vi "scan COM ports for XYZ stage.vi"(8 "error in (no error)":errorcluster) -> (0 "error out":errorcluster, 1 "Stage found?":bool, 2 "card type (F for old cards, T for new cards)":bool, 3 "VISA resource name out":refnum<visa-resource-name>)   [LabVIEW 2012]
uses:
  <vilib>/Instr/_visa.llb/VISA Flush IO Buffer Mask.ctl
  <vilib>/Instr/_visa.llb/VISA Find Search Mode.ctl
  <vilib>/Instr/_visa.llb/VISA Configure Serial Port (Instr).vi
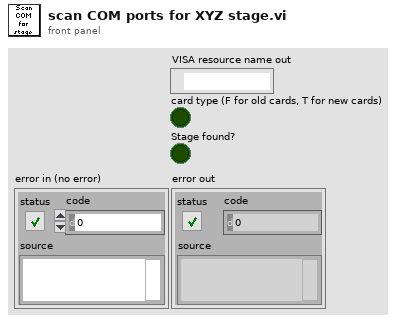
[diagram p1: front panel]
types:
  T1 = typedef "VISA Find Search Mode.ctl" = u32
  T2 = typedef "VISA Flush IO Buffer Mask.ctl" = u16
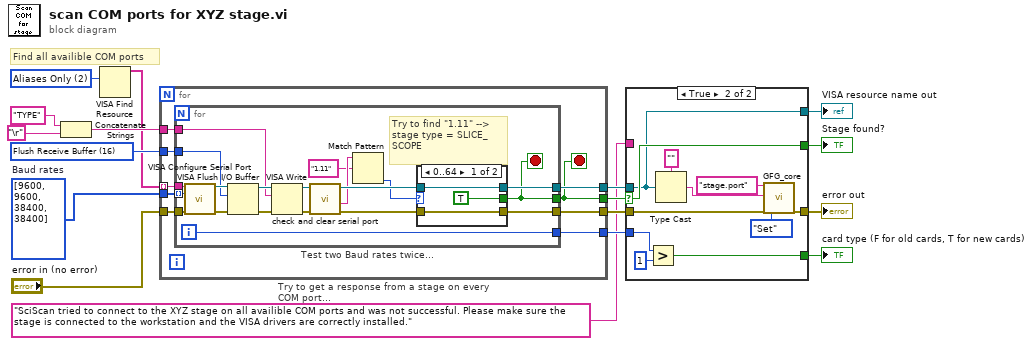
[diagram p0: block diagram]
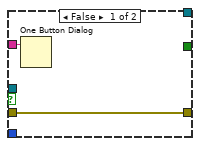
[diagram p2: hidden frame]
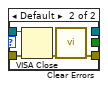
[diagram p3: hidden frame]
diagram:
  w13 = T1 2 items=["Canonical Names Only"=0, "Aliases Only"=2, "Include Matching Aliases"=3, "Include All Aliases"=4] ("Search Mode")
  w12 = u32[] [9600, 9600, 38400, 38400]  # Baud rates
  w16 = T2 16 items=["Flush Receive Buffer"=16, "Write Transmit Buffer to Device"=32, "Flush Receive Buffer (No I/O)"=64, "Flush Transmit Buffer"=128] ("Mask")
  # "Find all availible COM ports"
  n1 = Concatenate Strings("TYPE" ("write buffer"), "\r") -> (w14:string)
  n2 = VISA Find Resource(10:w13) -> (3:w11:string[])  [unwired: 2 in, 2 out]
  n3 = for "Try to get a response from a stage on every COM port..." {
    tunnel: w11 -> [w26] mode=indexing
    tunnel: w16 -> [w25]
    tunnel: w14 -> [w24]
    tunnel: w12 -> [w23]
    tunnel: [w22] -> w6
    tunnel: [w21] -> w5
    tunnel: [w20] -> w7
    tunnel: [w19] -> w9
    tunnel: "error in (no error)" -> [w18]
    stop <- w20 stop-if-true
    n4 = for "Test two Baud rates twice..." {
      tunnel: w26 -> [w40]
      tunnel: w25 -> [w37]
      tunnel: w24 -> [w36]
      tunnel: [w35] -> w22
      tunnel: [w34] -> w21
      tunnel: w23 -> [w33] mode=indexing
      tunnel: [w32] -> w19
      tunnel: [w31] -> w20
      tunnel: w18 -> [w30]
      i -> [w32]
      stop <- w31 stop-if-true
      # "Try to find \"1.11\" --> stage type = SLICE_SCOPE"
      n5 = call-poly "VISA Configure Serial Port"("VISA resource name"=w40, "baud rate (9600)"=w33, "error in (no error)"=w30) -> ("VISA resource name out"=w45:refnum<visa-resource-name>, "error out"=w46:errorcluster)  [unwired: 11 in]
      n6 = VISA Flush I/O Buffer(VISA resource name=w45, mask (16)=w37, error in (no error)=w46) -> (VISA resource name out=w39:refnum<visa-resource-name>, error out=w38:errorcluster)
      n7 = VISA Write(VISA resource name=w39, write buffer=w36, error in (no error)=w38) -> (VISA resource name out=w44:refnum<visa-resource-name>, error out=w43:errorcluster)  [unwired: 1 out]
      n8 = call "check and clear serial port.vi"("error in (no error)"=w43, "VISA resource name in"=w44) -> ("error out"=w41:errorcluster, "read buffer"=w28:string, "VISA resource name out"=w42:refnum<visa-resource-name>)  [unwired: 6 in, 1 out]
      n9 = Match Pattern(string=w28, regular expression="1.11" ("read buffer")) -> (offset past match=w29:i32)  [unwired: 1 in, 3 out]
      n10 = case shown="0..64" w29 {
        tunnel: w42 -> [w48 w53]
        tunnel: w41 -> [w49 w52]
        tunnel: [w49 w50] -> w34
        tunnel: [w48 _] -> w35
        tunnel: [TRUE _] -> w31
        frame 0..64 {
        }
        frame Default {
          n11 = VISA Close(VISA resource name=w53, error in (no error)=w52) -> (error out=w51:errorcluster)
          n12 = call <vilib>:"Clear Errors.vi"("error in (no error)"=w51) -> ("error out"=w50:errorcluster)  [unwired: 6 in]
        }
      }
    }
  }
  n13 = case shown="True" w7 {
    selector: w7 -> [_ w58]
    tunnel: [_ w65] -> w10
    tunnel: w9 -> [_ w64]
    tunnel: w6 -> [_ w57]
    tunnel: w5 -> [w54 w56]
    tunnel: "SciScan tried to connect to the XYZ stage on all availible COM ports and was not successful. Please make sure the stage is connected to the workstation and the VISA drivers are correctly installed." ("message") -> [w55 _]
    tunnel: [_ w58] -> w3
    tunnel: [_ w57] -> w2
    tunnel: [w54 w59] -> w1
    frame False {
      n14 = One Button Dialog(message=w55) -> ()  [unwired: 1 in, 1 out]
    }
    frame True {
      n15 = Greater?(x=w64, y=1) -> (0:w65:bool)
      n16 = Type Cast(type="" ("Variable Name in"), x=w57) -> (*(type *) &x=w61:string)
      n17 = call "GFG_core.vi"("Variable Name in"="stage.port", "Variant in"=w61, "error in (no error)"=w56, "Action"=enum16{"Init", "Set", "Get", "Clear"}."Set") -> ("error out"=w59:errorcluster)  [unwired: 9 in, 6 out]
    }
  }
  "card type (F for old cards, T for new cards)" <- w10
  "error out" <- w1
  "VISA resource name out" <- w2
  "Stage found?" <- w3
